vi "Up_PanelSetting.vi"() -> ()   [LabVIEW 2019]
uses:
  <vilib>/userdefined/High Color/IMAQdx.ctl
panel:
  in  "Up_Flg_Edit":refnum<vi>
  in  "Up_ProjectName":refnum<vi>
  in  "UpSystem_Path":path=path "C:/Users/Public/Documents/Vicomm"
  in  "UpSession In":T1="MV-CA060-10GC" caption="Up_Session In"
  in  "Up_Btn_Exist":refnum<vi>
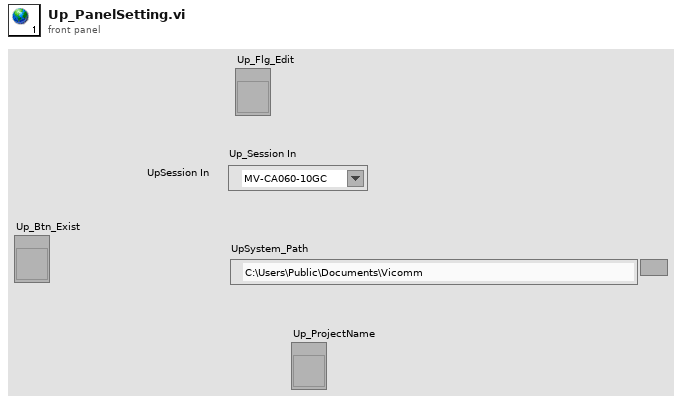
[diagram p1: front panel]
types:
  T1 = typedef "IMAQdx.ctl" = refnum<k21>
diagram:
